vi "CRYMain Window Menu Setting.vi"(11 "sAction":string) -> ()   [LabVIEW 2013]
uses:
  CRYProject/CRYProject Editor Global.vi
  CRYDocument/CRYReport Global.vi
  CRYMainGlobal.vi
  SubVI/CRYMain Sub Window Global.vi
panel:
  # "Main Menu State Setting"
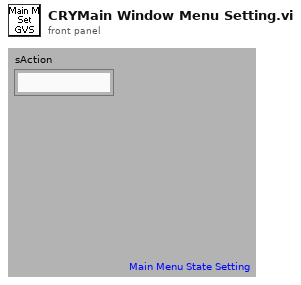
[diagram p1: front panel]
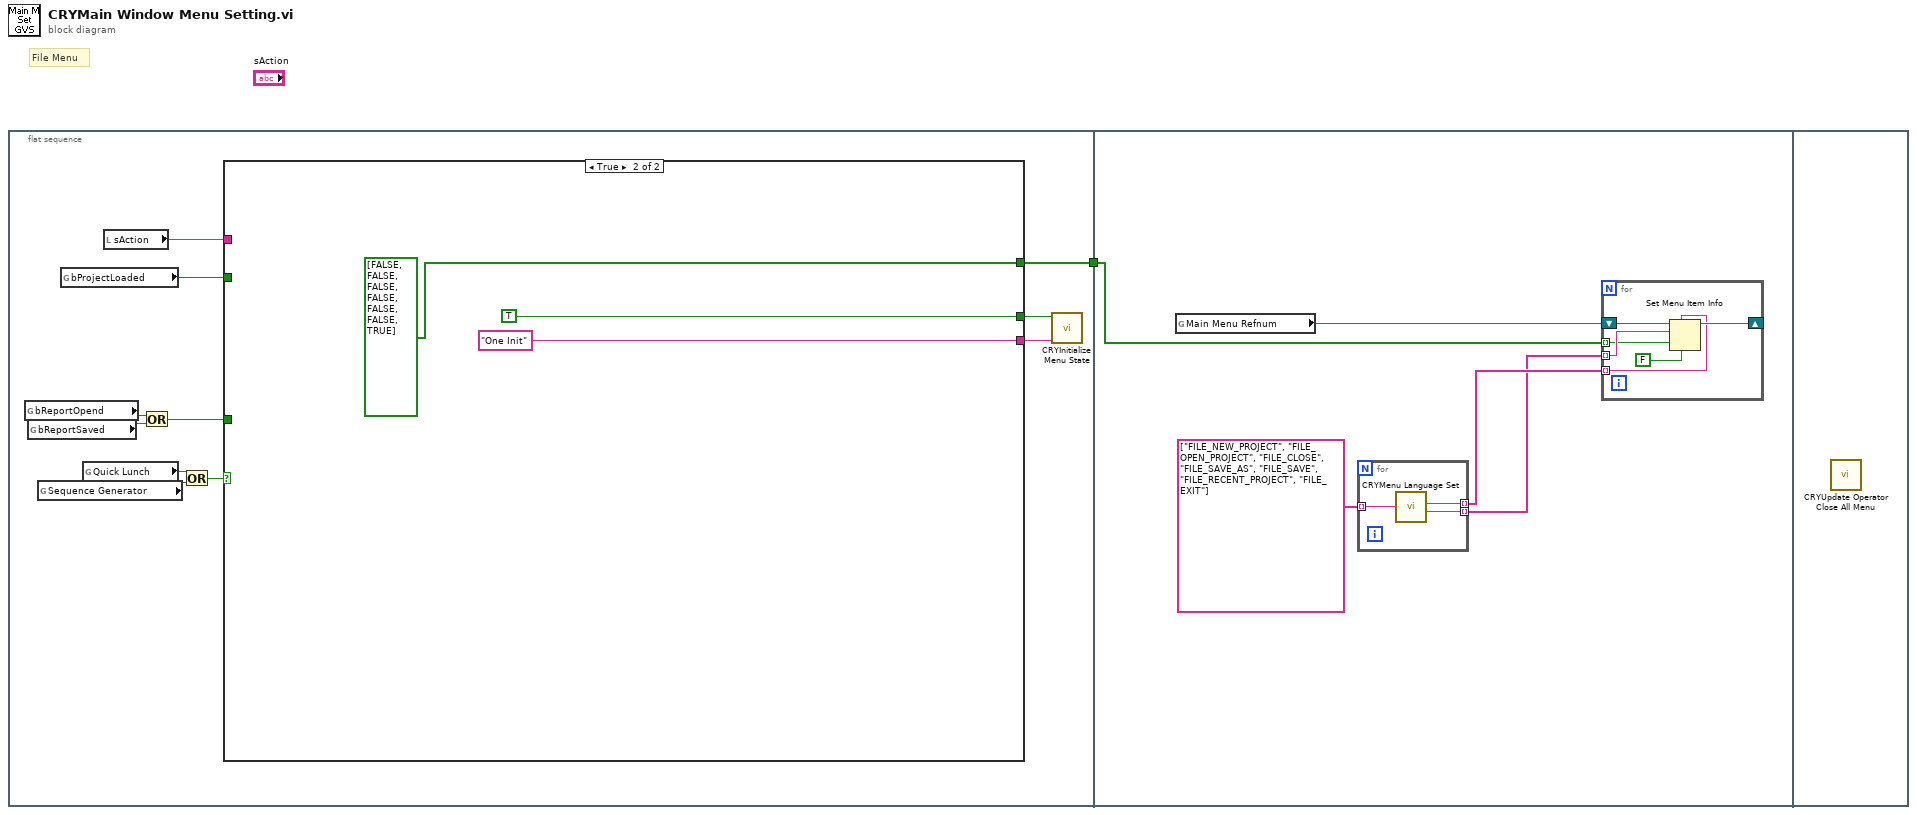
[diagram p0: block diagram]
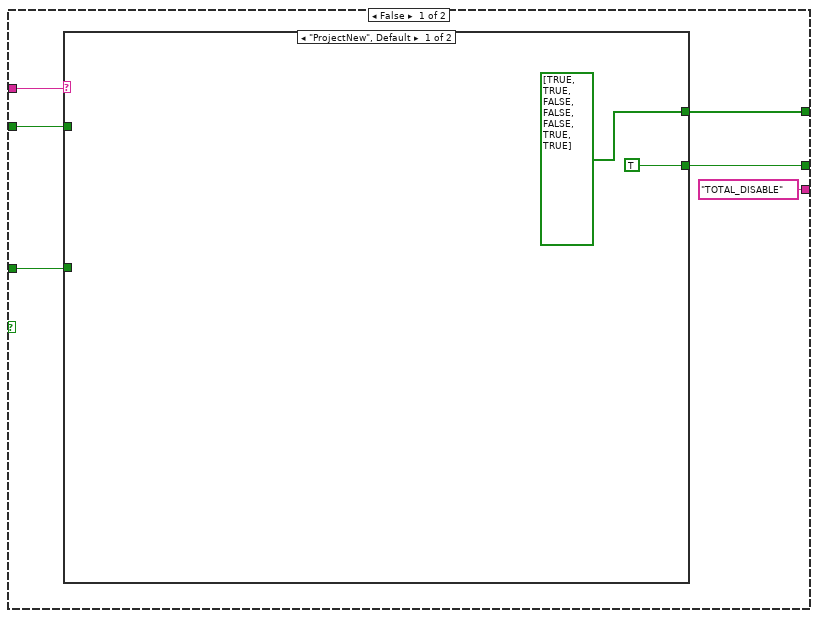
[diagram p2: hidden frame]
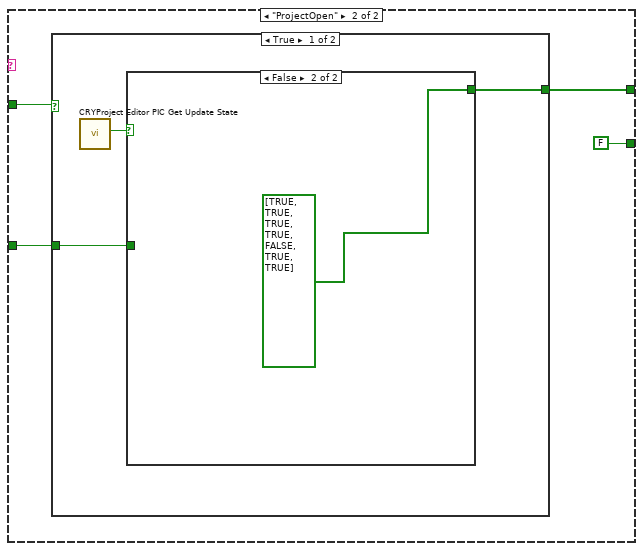
[diagram p3: hidden frame]
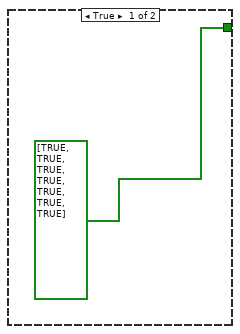
[diagram p4: hidden frame]
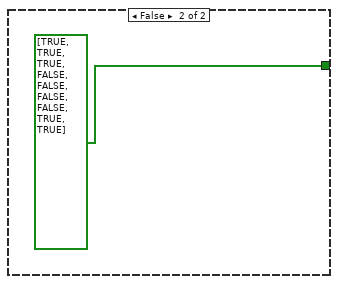
[diagram p5: hidden frame]
diagram:
  # "File Menu"
  n1 = flat-sequence {
    tunnel: [w12] -> w1
    tunnel: w1 -> [w34]
    frame #0 {
      n2 = global read "CRYReport Global.vi" "bReportOpend"() -> (w7:bool)
      n3 = global read "CRYReport Global.vi" "bReportSaved"() -> (w8:bool)
      n4 = global read "CRYMainGlobal.vi" "Sequence Generator"() -> (w3:bool)
      n5 = global read "CRYProject Editor Global.vi" "bProjectLoaded"() -> (w9:bool)
      n6 = global read "CRYMainGlobal.vi" "Quick Lunch"() -> (w4:bool)
      n7 = local read "sAction"() -> (w10:string)
      n8 = Or(x=w7, y=w8) -> (x .or. y?=w6:bool)
      n9 = Or(x=w4, y=w3) -> (x .or. y?=w2:bool)
      n10 = case shown="True" w2 {
        tunnel: [w18 bool[] [FALSE, FALSE, FALSE, FALSE, FALSE, FALSE, TRUE]] -> w12
        tunnel: [w17 TRUE ("enabled")] -> w11
        tunnel: w10 -> [w16 _]
        tunnel: w9 -> [w15 _]
        tunnel: w6 -> [w14 _]
        tunnel: ["TOTAL_DISABLE" ("sAction") "One Init" ("sAction")] -> w5
        frame False {
          n11 = case shown="\"ProjectNew\", Default" w16 {
            tunnel: [bool[] [TRUE, TRUE, FALSE, FALSE, FALSE, TRUE, TRUE] w24] -> w18
            tunnel: [TRUE ("enabled") FALSE ("enabled")] -> w17
            tunnel: w15 -> [_ w22]
            tunnel: w14 -> [_ w21]
            frame "ProjectNew", Default {
            }
            frame "ProjectOpen" {
              n12 = case shown="True" w22 {
                tunnel: [w27 bool[] [TRUE, TRUE, TRUE, FALSE, FALSE, FALSE, FALSE, TRUE, TRUE]] -> w24
                tunnel: w21 -> [w25 _]
                frame True {
                  n13 = call "CRYProject Editor PIC Get Update State.vi"() -> ("bChangeState"=w26:bool)  [unwired: 10 in, 1 out]
                  n14 = case shown="False" w26 {
                    tunnel: [bool[] [TRUE, TRUE, TRUE, TRUE, TRUE, TRUE, TRUE] bool[] [TRUE, TRUE, TRUE, TRUE, FALSE, TRUE, TRUE]] -> w27
                    tunnel: w25 -> [_ _]
                    frame True {
                    }
                    frame False {
                    }
                  }
                }
                frame False {
                }
              }
            }
          }
        }
        frame True {
        }
      }
      n15 = call "CRYInitialize Menu State.vi"("sAction"=w5, "Is Disable?"=w11) -> ()  [unwired: 10 out]
    }
    frame #1 {
      n16 = global read "CRYMain Sub Window Global.vi" "Main Menu Refnum"() -> (w35:refnum<k9>)
      n17 = for {
        tunnel: string[] ["FILE_NEW_PROJECT", "FILE_OPEN_PROJECT", "FILE_CLOSE", "FILE_SAVE_AS", "FILE_SAVE", "FILE_RECENT_PROJECT", "FILE_EXIT"] -> [w41] mode=indexing
        tunnel: [w40] -> w38 mode=indexing
        tunnel: [w39] -> w37 mode=indexing
        n18 = call "CRYMenu Language Set.vi"("sID"=w41) -> ("sMultibyte_Out"=w39:string, "sID_Out"=w40:string)  [unwired: 7 in, 2 out]
      }
      n19 = for {
        tunnel: w37 -> [w45] mode=indexing
        tunnel: w38 -> [w44] mode=indexing
        shift-right: [w46] -> _
        shift-left: w35 -> [w47]
        tunnel: w34 -> [w43] mode=indexing
        n20 = Set Menu Item Info(6:FALSE ("checked"), 7:w44, 9:w43, 10:w45, 11:w47) -> (3:w46:refnum<k9>)  [unwired: 1 in, 2 out]
      }
    }
    frame #2 {
      n21 = call "CRYUpdate Operator Close All Menu.vi"() -> ()  [unwired: 12 in]
    }
  }
